vi "imp_test_v7_2encoder.vi"() -> ()   [LabVIEW 2014]
uses:
  <vilib>/LabVIEW Targets/FPGA/cRIO/shared/nicrio_ModuleControls/nicrio_cRIO-9237_DataRatesRing.ctl
  <vilib>/LabVIEW Targets/FPGA/cRIO/shared/nicrio_ModuleControls/nicrio_cRIO-9237_ExcitationVoltageRing.ctl
  <vilib>/rvi/FXPMathLib/FxpSinAndCos/subVIs/nifxpmath_SinAndCos_SimConfig.ctl
  <vilib>/rvi/Emulation/niFpgaGetClockAttributes.vi
  <vilib>/rvi/Emulation/niFpgaSctlEmulationGetInTimedLoop.vi
  <vilib>/rvi/Emulation/niFpgaEmulationReportErrorSimple.vi
  <vilib>/rvi/Emulation/niFpgaProcessEmulError.vi
  <vilib>/rvi/interface/RandomDataEmulation/nirviRandomDataMultiElementFPGAFIFO.vi
  <instcachedir>/0/nirviRandomDataMultiElementFPGAFIFO_AD0CFC12EF974623A9C2E4184BC062B2.lvgen/nirviRandomDataMultiElementFPGAFIFO_AD0CFC12EF974623A9C2E4184BC062B2_023.vi
  <vilib>/rvi/interface/RandomDataEmulation/niFpgaRandomDataHandleErrors.vi
  <vilib>/rvi/Emulation/niFpgaCriticalErrorInLSC.vi
  <vilib>/rvi/eio/common/nirviEmuTemplateMethod_errors.vi
  <vilib>/rvi/FXPMathLib/FxpSinAndCos/simVIs/DllFxpSinAndCosTemp_sub.vi
  <vilib>/rvi/eio/common/nirviEmuTemplatePropertySet_errors.vi
  <vilib>/rvi/DataTransferAndStorage/Container/XNode/niFpgaContainer.xnode
  <vilib>/rvi/interface/RandomDataEmulation/nirviRandomDataFpgaMultiElementTemplate.vi
  <vilib>/eio/EIONode/EIONode.xnode
  <vilib>/rvi/FXPMathLib/FxpMul/XNode/nifxpmath_Multiplier.xnode
  <vilib>/rvi/FXPMathLib/FxpSinAndCos/XNode/nifxpmath_SinAndCos.xnode
  <vilib>/rvi/Analysis/measure/butterworth/XNode/niFpgaButterworthFilter.xnode
  <vilib>/rvi/FXPMathLib/FxpSub/XNode/nifxpmath_Sub.xnode
  <vilib>/rvi/FXPMathLib/FxpAdd/XNode/nifxpmath_Add.xnode
  <vilib>/eio/EIOPropertyNode/EIOPropertyNode.xnode
  <vilib>/rvi/eio/common/nirviEmuTemplatePropertyGet_errors.vi
  <vilib>/rvi/eio/common/nirviEmuTemplatePropertyGet_noerrors.vi
  <vilib>/rvi/eio/common/nirviEmuTemplatePropertySet_noerrors.vi
  <vilib>/rvi/FXPMathLib/sim/FxpSim.dll
panel:
  out "Encoder Position":i32
  out "rad_y (NrTheta)":fxp<+/-,33,20>
  out "D_y (mm)":fxp<+/-,32,7>
  in  "Encoder select":i16(ring) items=["Encoder", "Mag. encoder"]
  in  "Mag encoder coeff.":fxp<+/-,32,14>
  in  "Strain selection_y":i16(ring) items=["Raw", "Avg.8", "Avg.8 w. filter"]
  in  "Belt_oy":fxp<+/-,7,7>
  in  "Belt_my":fxp<+/-,6,6>
  out "Fp_dc":fxp<+/-,32,10>
  out "Fy_dc":fxp<+/-,32,10>
  in  "Zero_y":bool
  in  "Zero_p":bool
  in  "S/F coeff_p":fxp<+/-,25,-10>
  in  "S/F coeff_y":fxp<+/-,25,-10>
  out "Force_p":fxp<+/-,32,10>
  in  "Strain selection_p":i16(ring) items=["Raw", "Avg.8", "Avg.8 w. filter"]
  out "Strain_p (Avg8 w. f)":fxp<+/-,36,8>
  in  "Strain_p Avg.8 coeff.":i32[](array[numeric])=[946630756, 63555534]
  out "Strain_p (Avg8)":fxp<+/-,36,4>
  out "Raw Strain_p":fxp<+/-,36,4>
  out "Mod6/AI3":fxp<+/-,36,4>
  in  "Strain gage reset_p":bool
  out "rad_ym":fxp<+/-,33,20>
  out "D_ym":fxp<+/-,32,7>
  out "encoder position_ym":i32
  in  "Encoder reset_p":bool
  out "Strain_y (Avg8 w. f)":fxp<+/-,36,8>
  in  "Strain_y Avg8 coeff.":i32[](array[numeric])=[-898916953, 1957103773, 3888751]
  out "Dyr_for":fxp<+/-,22,7>
  in  "Command_y":i16(ring) items=["Step", "Sine"]
  out "Strain_y (Avg8)":fxp<+/-,36,4>
  out "vb_y":fxp<+/-,38,8>
  out "va_y":fxp<+/-,38,8>
  out "fyt_d":fxp<+/-,36,18>
  out "Fr_y":fxp<+/-,32,10>
  in  "Bv_y":fxp<+/-,22,8>
  out "Dy_error_dd":fxp<+/-,36,16>
  out "Dy_error_d":fxp<+/-,33,8>
  in  "Kv_y":fxp<+/-,22,8>
  out "Dy_error":fxp<+/-,22,7>
  out "Dyr_sin_dd":fxp<+/-,35,20>
  out "Dyr_sin_d":fxp<+/-,33,15>
  out "Sin omega_y":fxp<+/-,34,9>
  out "Dyr_sin":fxp<+/-,22,7>
  in  "Sin offset_y":fxp<+/-,22,7>
  in  "Sin magnitude_y":fxp<+/-,21,6>
  out "Time now(s)":fxp<+,52,14>
  in  "Sin wave freq._y (Hz)":fxp<+/-,32,6>
  in  "Dyr_step":fxp<+/-,22,7>
  in  "Drive mode":i16(ring) items=["Backward", "Forward"]
  out "Dy_dd":fxp<+/-,36,25>
  in  "Dy_dd coeff.":i32[](array[numeric])=[946630756, 63555534]
  out "dFy_PID":fxp<+/-,36,18>
  in  "dFy_PID coeff.":i32[](array[numeric])=[946630756, 63555534]
  out "fyt_i":fxp<+/-,36,16>
  out "Fy_PID":fxp<+/-,36,16>
  in  "fy_tolorance":fxp<+,22,6>
  in  "Ki_y":fxp<+/-,36,9>
  in  "Kd_y":fxp<+/-,36,9>
  out "fy_tilde":fxp<+/-,32,10>
  in  "Kp_y":fxp<+/-,36,9>
  out "vq_y_F":fxp<+/-,20,5> format="%.57g"
  out "vd_y_F":fxp<+/-,20,5>
  in  "dFy_add":bool
  in  "Stop motor_y":bool
  out "Dy_d (mm/s)":fxp<+/-,36,11>
  out "omega_y (rad/s)":fxp<+/-,20,9>
  in  "mt0_omega_y":u32
  out "mt_omega_y":u32
  out "rad_y":fxp<+/-,33,20>
  out "D_y":fxp<+/-,32,7>
  out "encoder position_y":i32
  in  "Encoder reset_y":bool
  in  "Ini coe.":bool
  out "Loop rate (kHz)":fxp<+/-,36,7>
  out "Force_y":fxp<+/-,32,10>
  out "Raw Strain_y":fxp<+/-,36,4>
  in  "Strain gage reset_y":bool
  in  "Stop (Strain)":bool
  out "Mod6/AI2":fxp<+/-,36,4>
  in  "Excitation Voltage":T1 items=["2.5 Volts", "3.3 Volts", "5.0 Volts", "10.0 Volts", "External Excitation"]
  in  "Data Rate":T2=1 items=["50.000 kS/s (NI 9237)"=1, "25.000 kS/s (NI 9237)"=2, "16.667 kS/s (NI 9237)"=3, "12.500 kS/s (NI 9237)"=4, "10.000 kS/s (NI 9237)"=5, "8.333 kS/s (NI 9237)"=6, "7.143 kS/s (NI 9237)"=7, "6.250 kS/s (NI 9237)"=8, "5.556 kS/s (NI 9237)"=9, "5.000 kS/s (NI 9237)"=10, "4.545 kS/s (NI 9237)"=11, "4.167 kS/s (NI 9237)"=12, "3.846 kS/s (NI 9237)"=13, "3.571 kS/s (NI 9237)"=14, "3.333 kS/s (NI 9237)"=15, "3.125 kS/s (NI 9237)"=16, "2.941 kS/s (NI 9237)"=17, "2.778 kS/s (NI 9237)"=18, "2.632 kS/s (NI 9237)"=19, "2.500 kS/s (NI 9237)"=20, "2.381 kS/s (NI 9237)"=21, "2.273 kS/s (NI 9237)"=22, "2.174 kS/s (NI 9237)"=23, "2.083 kS/s (NI 9237)"=24, "2.000 kS/s (NI 9237)"=25, "1.923 kS/s (NI 9237)"=26, "1.852 kS/s (NI 9237)"=27, "1.786 kS/s (NI 9237)"=28, "1.724 kS/s (NI 9237)"=29, "1.667 kS/s (NI 9237)"=30, "1.613 kS/s (NI 9237)"=31]
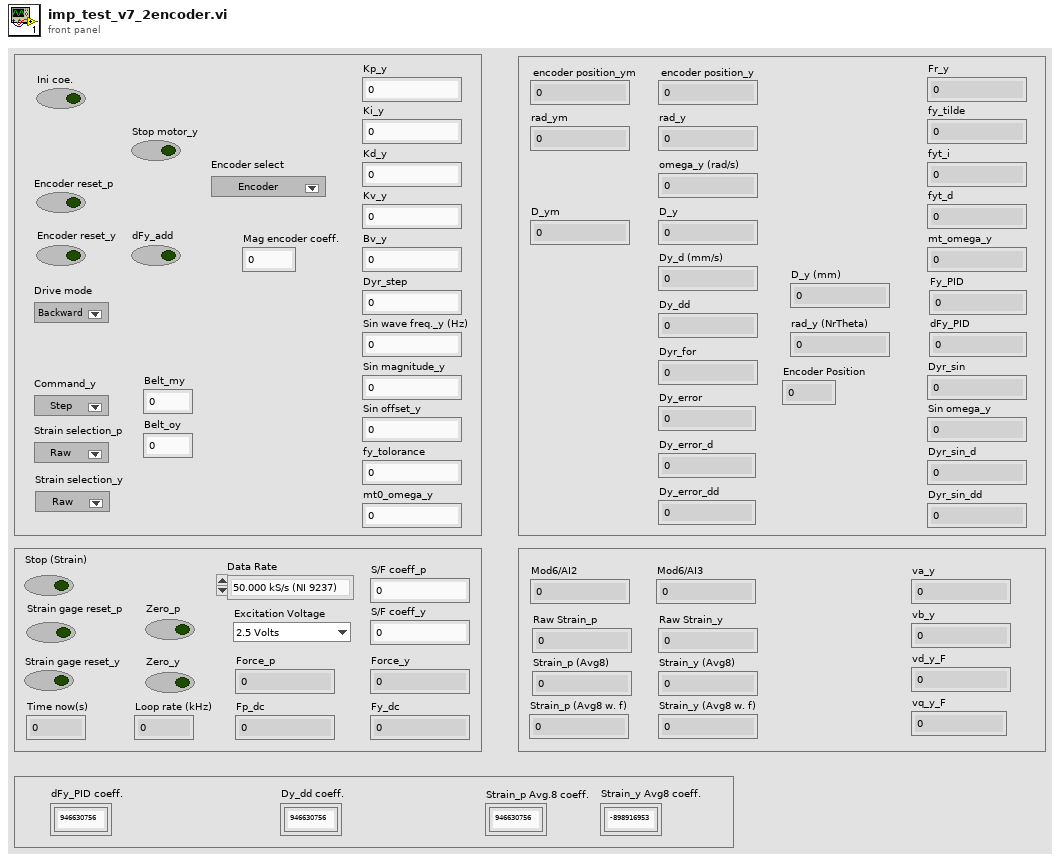
[diagram p1: front panel]
types:
  T1 = typedef "nicrio_cRIO-9237_ExcitationVoltageRing.ctl" = u8
  T2 = typedef "nicrio_cRIO-9237_DataRatesRing.ctl" = u8
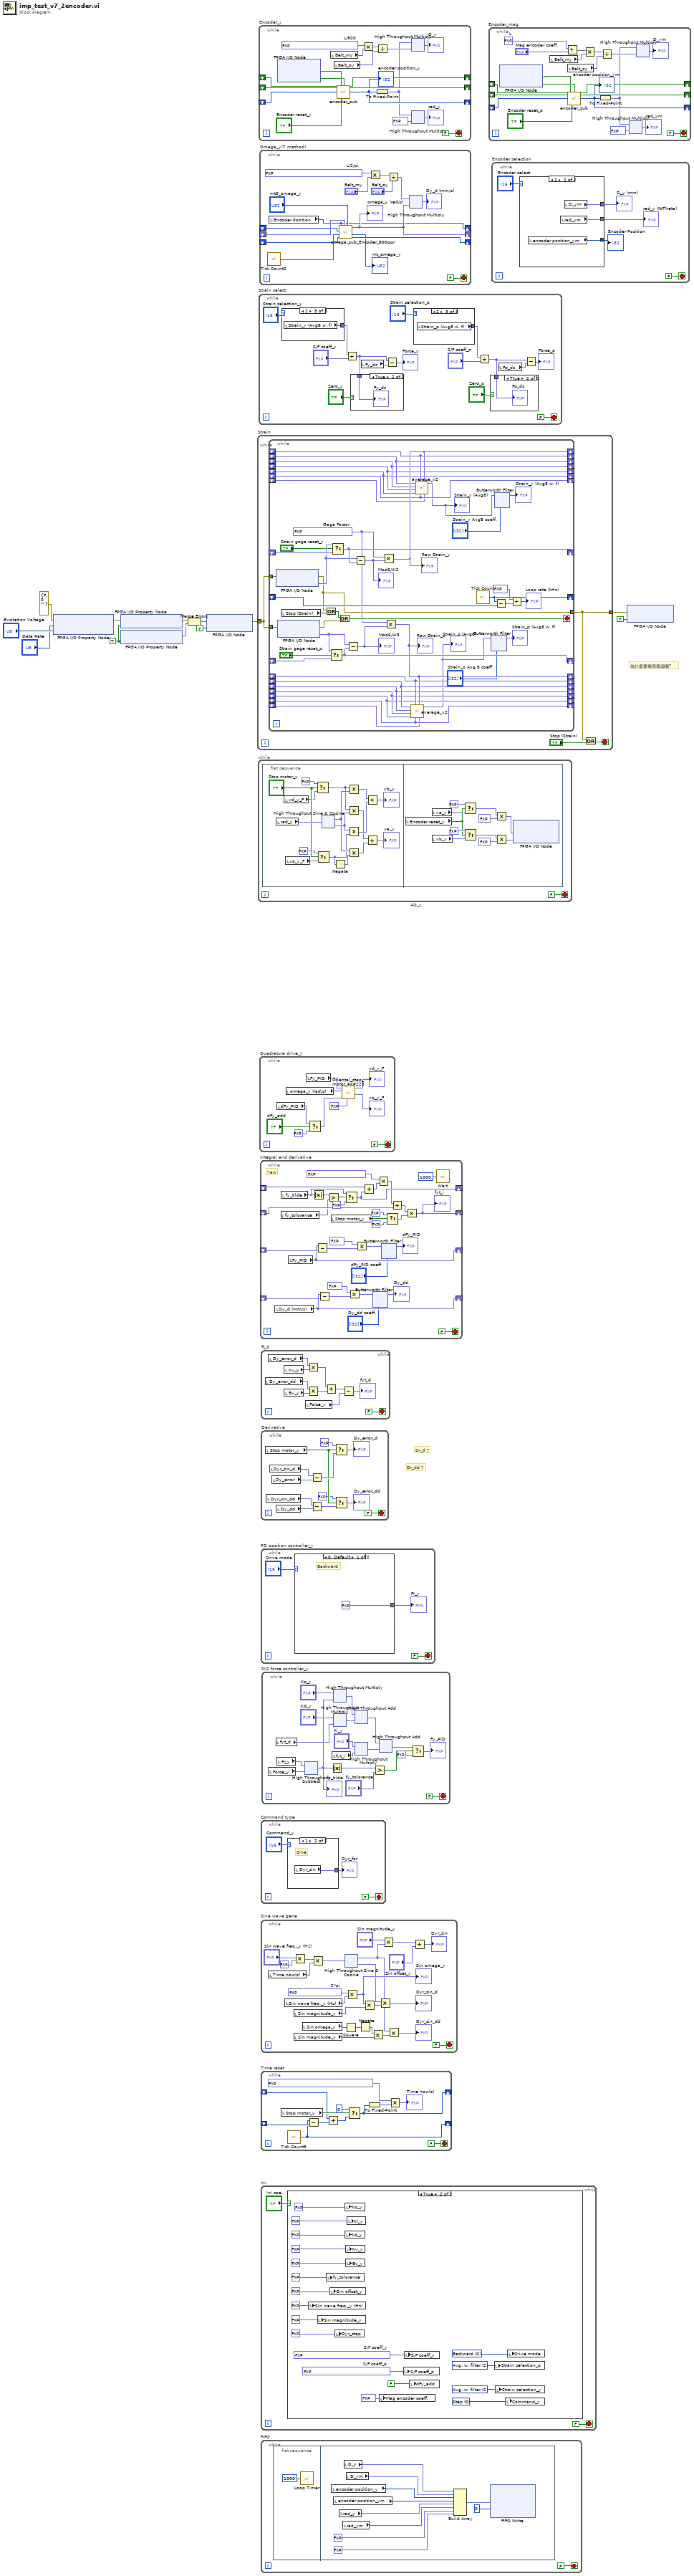
[diagram p0: block diagram]
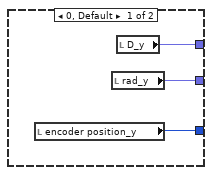
[diagram p2: hidden frame]
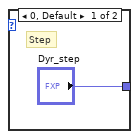
[diagram p3: hidden frame]
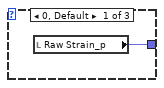
[diagram p6: hidden frame]
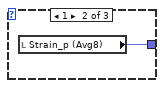
[diagram p7: hidden frame]
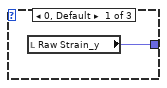
[diagram p8: hidden frame]
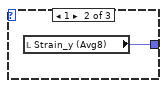
[diagram p9: hidden frame]
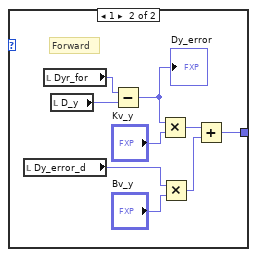
[diagram p10: hidden frame]
diagram:
  w5 = TRUE ("Half-Bridge Enable")
  # "為什麼要寫兩個迴圈?"
  # "Dr_dd ?"
  # "Dr_d ?"
  n1 = xnode "FPGA I/O Property Node"("error in"=errorcluster {"status"=FALSE, "code"=0, "source"=""}, "Data Rate"="Data Rate", "Excitation Voltage"="Excitation Voltage") -> ("error out"=w10:errorcluster)  [unwired: 1 in, 1 out]
  n2 = xnode "FPGA I/O Property Node"("error in"=w10, "Half-Bridge Enable"=w5) -> ("error out"=w3:errorcluster)  [unwired: 1 in, 1 out]
  n3 = xnode "FPGA I/O Property Node"("Half-Bridge Enable"=w5) -> ("error out"=w2:errorcluster)  [unwired: 2 in, 1 out]
  n4 = Merge Errors(w3, w2) -> (w4:errorcluster)
  n5 = xnode "FPGA I/O Node"("error in"=w4, "Mod6/Start"=TRUE) -> ("error out"=w8:errorcluster)  [unwired: 1 in, 1 out]
  n6 = while "Strain" {
    tunnel: w8 -> [w15]
    tunnel: [w13] -> w1
    stop <- w14 stop-if-true
    n7 = while {
      tunnel: w15 -> [w61]
      tunnel: [w34] -> w13
      shift-right: [w58] -> _
      shift-left: _ -> [w59]
      shift-right: [w54] -> _
      shift-left: _ -> [w55]
      shift-right: [w49] -> _
      shift-left: _ -> [w48]
      shift-right: [w48] -> _
      shift-left: _ -> [w47]
      shift-right: [w47] -> _
      shift-left: _ -> [w46]
      shift-right: [w46] -> _
      shift-left: _ -> [w45]
      shift-right: [w45] -> _
      shift-left: _ -> [w44]
      shift-right: [w44] -> _
      shift-left: _ -> [w43]
      shift-right: [w43] -> _
      shift-left: _ -> [w42]
      tunnel: w15 -> [w38]
      shift-right: [w31] -> _
      shift-left: _ -> [w32]
      shift-right: [w27] -> _
      shift-left: _ -> [w26]
      shift-right: [w26] -> _
      shift-left: _ -> [w25]
      shift-right: [w25] -> _
      shift-left: _ -> [w24]
      shift-right: [w24] -> _
      shift-left: _ -> [w23]
      shift-right: [w23] -> _
      shift-left: _ -> [w22]
      shift-right: [w22] -> _
      shift-left: _ -> [w21]
      shift-right: [w21] -> _
      shift-left: _ -> [w20]
      stop <- w35 stop-if-true
      w29 = fxp<+,20,2> 2.115001678466797  # Gage Factor
      n8 = xnode "FPGA I/O Node"("error in"=w61) -> ("error out"=w34:errorcluster, "Mod6/AI2"=w56:fxp<+/-,24,-4>)  [unwired: 1 in, 1 out]
      n9 = xnode "FPGA I/O Node"("error in"=w38) -> ("error out"=w36:errorcluster, "Mod6/AI3"=w30:fxp<+/-,24,-4>)  [unwired: 1 in, 1 out]
      n10 = local read "Stop (Strain)"() -> (w60:bool)
      n11 = Or(x=w34, y=w60) -> (x .or. y?=w37:bool)
      n12 = Select(t=w30, s="Strain gage reset_p", f=w32) -> (s? t:f=w31:fxp<+/-,24,-4>)
      n13 = Select(t=w56, s="Strain gage reset_y", f=w59) -> (s? t:f=w58:fxp<+/-,24,-4>)
      n14 = Or(x=w37, y=w36) -> (x .or. y?=w35:bool)
      n15 = Subtract(x=w30, y=w31) -> (x-y=w28:fxp<+/-,30,-3>)
      "Mod6/AI3" <- w28
      n16 = Subtract(x=w56, y=w58) -> (x-y=w57:fxp<+/-,30,-3>)
      "Mod6/AI2" <- w57
      n17 = Multiply(x=w29, y=w57) -> (x*y=w49:fxp<+/-,41,6>)
      "Raw Strain_y" <- w49
      n18 = Multiply(x=w29, y=w28) -> (x*y=w27:fxp<+/-,50,-1>)
      "Raw Strain_p" <- w27
      n19 = call "average_v2.vi"("Numeric 8"=w20, "Numeric"=w27, "Numeric 7"=w21, "Numeric 2"=w26, "Numeric 6"=w22, "Numeric 5"=w23, "Numeric 4"=w24, "Numeric 3"=w25) -> ("Mean (8pt)"=w19:fxp<+/-,32,4>)  [unwired: 1 in, 2 out]
      "Strain_p (Avg8)" <- w19
      n20 = call "average_v2.vi"("Numeric 8"=w42, "Numeric"=w49, "Numeric 7"=w43, "Numeric 2"=w48, "Numeric 6"=w44, "Numeric 5"=w45, "Numeric 4"=w46, "Numeric 3"=w47) -> ("Mean (8pt)"=w41:fxp<+/-,32,4>)  [unwired: 1 in, 2 out]
      "Strain_y (Avg8)" <- w41
      n21 = call "Tick Count"() -> ("Tick Count(uSec)"=w54:u32)
      n22 = xnode "Butterworth Filter"("input data"=w19, "scaled coefficients"="Strain_p Avg.8 coeff.") -> ("output data"=→"Strain_p (Avg8 w. f)":fxp<+/-,36,8>)  [unwired: 1 in]
      n23 = xnode "Butterworth Filter"("input data"=w41, "scaled coefficients"="Strain_y Avg8 coeff.") -> ("output data"=→"Strain_y (Avg8 w. f)":fxp<+/-,32,4>)  [unwired: 1 in]
      n24 = Subtract(x=w54, y=w55) -> (x-y=w52:fxp<+/-,32,16>)
      n25 = Divide(x=fxp<+,7,10> 1000.0, y=w52) -> (x/y=→"Loop rate (kHz)":fxp<+/-,40,27>)
    }
    n26 = Or(x=w13, y="Stop (Strain)") -> (x .or. y?=w14:bool)
  }
  n27 = while "AO_y" {
    stop <- FALSE stop-if-true
    n28 = flat-sequence {
      frame #0 {
        n29 = local read "rad_y"() -> (w95:fxp<+/-,33,20>)
        n30 = local read "vd_y_F"() -> (w93:fxp<+/-,20,5>)
        n31 = local read "vq_y_F"() -> (w92:fxp<+/-,20,5>)
        n32 = Select(t=fxp<+/-,20,5> 0.0, s="Stop motor_y", f=w93) -> (s? t:f=w87:fxp<+/-,20,5>)
        n33 = Select(t=fxp<+/-,20,5> 0.0, s="Stop motor_y", f=w92) -> (s? t:f=w86:fxp<+/-,20,5>)
        n34 = xnode "High Throughput Sine & Cosine"("x (pi)"=w95) -> ("sin(x)"=w89:fxp<+/-,17,2>, "cos(x)"=w88:fxp<+/-,17,2>)
        n35 = Negate(x=w86) -> (-x=w85:fxp<+/-,21,6>)
        n36 = Multiply(x=w87, y=w89) -> (x*y=w84:fxp<+/-,37,7>)
        n37 = Multiply(x=w87, y=w88) -> (x*y=w82:fxp<+/-,37,7>)
        n38 = Multiply(x=w88, y=w86) -> (x*y=w83:fxp<+/-,37,7>)
        n39 = Multiply(x=w89, y=w85) -> (x*y=w81:fxp<+/-,36,6>)
        n40 = Add(x=w84, y=w83) -> (x+y=→"vb_y":fxp<+/-,38,8>)
        n41 = Add(x=w82, y=w81) -> (x+y=→"va_y":fxp<+/-,37,7>)
      }
      frame #1 {
        n42 = local read "Encoder reset_y"() -> (w128:bool)
        n43 = local read "va_y"() -> (w127:fxp<+/-,38,8>)
        n44 = local read "vb_y"() -> (w126:fxp<+/-,38,8>)
        n45 = Select(t=fxp<+,2,2> 3.0, s=w128, f=w127) -> (s? t:f=w132:fxp<+/-,38,8>)
        n46 = Select(t=fxp<+,1,1> 0.0, s=w128, f=w126) -> (s? t:f=w131:fxp<+/-,38,8>)
        n47 = Multiply(x=w132, y=fxp<+/-,1,0> -0.5) -> (x*y=w135:fxp<+/-,39,8>)
        n48 = Multiply(x=w131, y=fxp<+/-,1,0> -0.5) -> (x*y=w136:fxp<+/-,37,6>)
        n49 = xnode "FPGA I/O Node"("Mod8/AO2"=w135, "Mod8/AO3"=w136) -> ()  [unwired: 2 in, 2 out]
      }
    }
  }
  n50 = while "Strain select." {
    stop <- FALSE stop-if-true
    n51 = case shown="2" "Strain selection_y" {
      tunnel: [w157 w158 w159] -> w151
      frame 0, Default {
        n52 = local read "Raw Strain_y"() -> (w157:fxp<+/-,36,4>)
      }
      frame 1 {
        n53 = local read "Strain_y (Avg8)"() -> (w158:fxp<+/-,36,4>)
      }
      frame 2 {
        n54 = local read "Strain_y (Avg8 w. f)"() -> (w159:fxp<+/-,36,8>)
      }
    }
    n55 = Divide(x=w151, y="S/F coeff_y") -> (x/y=w144:fxp<+/-,32,10>)
    n56 = case shown="True" "Zero_y" {
      tunnel: w144 -> [_ w153]
      frame False {
      }
      frame True {
        "Fy_dc" <- w153
      }
    }
    n57 = local read "Fy_dc"() -> (w145:fxp<+/-,32,10>)
    n58 = Subtract(x=w144, y=w145) -> (x-y=→"Force_y":fxp<+/-,33,11>)
    n59 = case shown="2" "Strain selection_p" {
      tunnel: [w154 w155 w156] -> w149
      frame 0, Default {
        n60 = local read "Raw Strain_p"() -> (w154:fxp<+/-,36,4>)
      }
      frame 1 {
        n61 = local read "Strain_p (Avg8)"() -> (w155:fxp<+/-,36,4>)
      }
      frame 2 {
        n62 = local read "Strain_p (Avg8 w. f)"() -> (w156:fxp<+/-,36,8>)
      }
    }
    n63 = Divide(x=w149, y="S/F coeff_p") -> (x/y=w141:fxp<+/-,32,10>)
    n64 = case shown="True" "Zero_p" {
      tunnel: w141 -> [_ w152]
      frame False {
      }
      frame True {
        "Fp_dc" <- w152
      }
    }
    n65 = local read "Fp_dc"() -> (w139:fxp<+/-,32,10>)
    n66 = Subtract(x=w141, y=w139) -> (x-y=→"Force_p":fxp<+/-,33,11>)
  }
  n67 = while "Encoder_y" {
    shift-right: [w175] -> _
    shift-left: _ -> [w176]
    shift-right: [w177] -> _
    shift-left: _ -> [w178]
    shift-right: [w170] -> _
    shift-left: _ -> [w174]
    stop <- FALSE stop-if-true
    w164 = fxp<+/-,20,-5> 0.002499997615814209  # L/800
    n68 = xnode "FPGA I/O Node"() -> ("Mod4/DI3"=w173:bool, "Mod4/DI4"=w172:bool)  [unwired: 2 in, 2 out]
    n69 = local read "Belt_my"() -> (w163:fxp<+/-,6,6>)
    n70 = local read "Belt_oy"() -> (w161:fxp<+/-,7,7>)
    n71 = call "encoder_sub.vi"("A_pre"=w176, "B_pre"=w178, "Encoder Position_pre"=w174, "A input"=w173, "Encoder Position Reset"="Encoder reset_y", "B input"=w172) -> ("A"=w175:bool, "B"=w177:bool, "Encoder Position (Counts)"=w170:i32)  [unwired: 19 in]
    "encoder position_y" <- w170
    n72 = Multiply(x=w164, y=w163) -> (x*y=w162:fxp<+/-,26,1>)
    n73 = To Fixed-Point(number=w170) -> (fixed-point=w169:fxp<+/-,32,32>)  [unwired: 1 in]
    n74 = Divide(x=w162, y=w161) -> (x/y=w160:fxp<+/-,33,1>)
    n75 = xnode ("High Throughput Multiply")("x"=w169, "y"=w160) -> ("x*y"=→"D_y":fxp<+/-,64,33>)
    n76 = xnode ("High Throughput Multiply")("x"=w169, "y"=fxp<+/-,16,1> 0.125) -> ("x*y"=→"rad_y":fxp<+/-,48,33>)
  }
  n77 = while "Omega_y(T method)" {
    shift-right: [w185] -> _
    shift-left: _ -> [w186]
    shift-right: [w188] -> _
    shift-left: _ -> [w190]
    shift-right: [w192] -> _
    shift-left: _ -> [w193]
    stop <- FALSE stop-if-true
    w183 = fxp<+/-,32,0> 0.3183098859153688  # L/2/pi
    n78 = call "Tick Count2"() -> ("Tick Count(Ticks)"=w194:u32)
    n79 = local read "Encoder Position"() -> (w185:i32)
    n80 = call "omega_sub_Encoder_800ppr.vi"("mt0"="mt0_omega_y", "omega_pre"=w190, "ticks_m_pre"=w193, "ticks"=w194, "count_pre"=w186, "count"=w185) -> ("ticks_m"=w192:u32, "mt"=→"mt_omega_y":u32, "omega"=w188:fxp<+/-,20,9>)  [unwired: 3 in]
    "omega_y (rad/s)" <- w188
    n81 = Multiply(x=w183, y="Belt_my") -> (x*y=w181:fxp<+/-,38,6>)
    n82 = Divide(x=w181, y="Belt_oy") -> (x/y=w179:fxp<+/-,20,1>)
    n83 = xnode ("High Throughput Multiply")("x"=w179, "y"=w188) -> ("x*y"=→"Dy_d (mm/s)":fxp<+/-,40,10>)
  }
  n84 = while "Quadrature drive_y" {
    stop <- FALSE stop-if-true
    n85 = local read "dFy_PID"() -> (w196:fxp<+/-,36,18>)
    n86 = local read "omega_y (rad/s)"() -> (w204:fxp<+/-,20,9>)
    n87 = local read "Fy_PID"() -> (w197:fxp<+/-,36,16>)
    n88 = Select(t=w196, s="dFy_add", f=fxp<+,1,1> 0.0) -> (s? t:f=w200:fxp<+/-,36,18>)
    n89 = call "Oriental_step_motor_PKP225.vi"("F_Threshold"=fxp<+,12,12> 10.0, "dFmr"=w200, "omega"=w204, "Fmr"=w197) -> ("vq_F"=→"vq_y_F":fxp<+/-,20,5>, "vd_F"=→"vd_y_F":fxp<+/-,20,5>)  [unwired: 6 in]
  }
  n90 = while "Integral and derivative" {
    shift-right: [w229] -> _
    shift-left: _ -> [w228]
    shift-right: [w221] -> _
    shift-left: _ -> [w220]
    shift-right: [w231] -> _
    shift-left: _ -> [w232]
    shift-right: [w211] -> _
    shift-left: _ -> [w210]
    stop <- FALSE stop-if-true
    # "Yaw"
    n91 = local read "Dy_d (mm/s)"() -> (w211:fxp<+/-,36,11>)
    n92 = local read "fy_tolorance"() -> (w207:fxp<+,22,6>)
    n93 = local read "fy_tilde"() -> (w233:fxp<+/-,32,10>)
    n94 = local read "Fy_PID"() -> (w231:fxp<+/-,36,16>)
    n95 = Absolute Value(x=w233) -> (abs(x)=w235:fxp<+,32,10>)
    n96 = Subtract(x=w231, y=w232) -> (x-y=w219:fxp<+/-,37,17>)
    n97 = Subtract(x=w211, y=w210) -> (x-y=w213:fxp<+/-,36,11>)
    n98 = Greater?(x=w235, y=w207) -> (0:w236:bool)
    n99 = local read "Stop motor_y"() -> (w222:bool)
    n100 = Select(t=w233, s=w236, f=fxp<+/-,33,11> 0.0) -> (s? t:f=w229:fxp<+/-,33,11>)
    n101 = Multiply(x=fxp<+,7,10> 1000.0, y=w213) -> (x*y=w212:fxp<+/-,36,21>)
    n102 = Multiply(x=fxp<+,7,10> 1000.0, y=w219) -> (x*y=w216:fxp<+/-,32,18>)
    n103 = Add(x=w228, y=w229) -> (x+y=w234:fxp<+/-,34,12>)
    n104 = xnode "Butterworth Filter"("input data"=w212, "scaled coefficients"="Dy_dd coeff.") -> ("output data"=→"Dy_dd":fxp<+/-,36,25>)  [unwired: 1 in]
    n105 = Multiply(x=fxp<+/-,30,12> 0.000499725341796875, y=w234) -> (x*y=w227:fxp<+/-,34,10>)
    n106 = xnode "Butterworth Filter"("input data"=w216, "scaled coefficients"="dFy_PID coeff.") -> ("output data"=→"dFy_PID":fxp<+/-,36,22>)  [unwired: 1 in]
    n107 = Select(t=fxp<+,1,1> 0.0, s=w222, f=fxp<+,1,1> 1.0) -> (s? t:f=w225:fxp<+,1,1>)
    n108 = Add(x=w227, y=w220) -> (x+y=w226:fxp<+/-,36,16>)
    n109 = Multiply(x=w226, y=w225) -> (x*y=w221:fxp<+/-,34,18>)
    "fyt_i" <- w221
    n110 = call "Wait"("Count(uSec)"=u32 1000) -> ()  [unwired: 1 out]
  }
  n111 = while "PD position controller_y" {
    stop <- FALSE stop-if-true
    n112 = case shown="0, Default" "Drive mode" {
      tunnel: [fxp<+/-,62,19> 0.0 w259] -> w255
      frame 0, Default {
        # "Backward"
      }
      frame 1 {
        # "Forward"
        n113 = local read "Dy_error_d"() -> (w261:fxp<+/-,33,8>)
        n114 = local read "Dyr_for"() -> (w258:fxp<+/-,22,7>)
        n115 = local read "D_y"() -> (w266:fxp<+/-,32,7>)
        n116 = Subtract(x=w258, y=w266) -> (x-y=w265:fxp<+/-,33,8>)
        "Dy_error" <- w265
        n117 = Multiply(x=w265, y="Kv_y") -> (x*y=w263:fxp<+/-,54,15>)
        n118 = Multiply(x=w261, y="Bv_y") -> (x*y=w260:fxp<+/-,55,16>)
        n119 = Add(x=w263, y=w260) -> (x+y=w259:fxp<+/-,55,16>)
      }
    }
    "Fr_y" <- w255
  }
  n120 = while "Command type" {
    stop <- FALSE stop-if-true
    n121 = case shown="1" "Command_y" {
      tunnel: ["Dyr_step" w271] -> w268
      frame 0, Default {
        # "Step"
      }
      frame 1 {
        # "Sine"
        n122 = local read "Dyr_sin"() -> (w271:fxp<+/-,22,7>)
      }
    }
    "Dyr_for" <- w268
  }
  n123 = while "Sine wave gene" {
    stop <- FALSE stop-if-true
    w286 = fxp<+,20,3> 6.2831878662109375  # 2*pi
    n124 = local read "Time now(s)"() -> (w292:fxp<+,52,14>)
    n125 = local read "Sin wave freq._y (Hz)"() -> (w285:fxp<+/-,32,6>)
    n126 = Multiply(x="Sin wave freq._y (Hz)", y=fxp<+/-,10,3> 2.0) -> (x*y=w293:fxp<+/-,41,9>)
    n127 = local read "Sin magnitude_y"() -> (w283:fxp<+/-,21,6>)
    n128 = local read "Sin magnitude_y"() -> (w276:fxp<+/-,21,6>)
    n129 = local read "Sin omega_y"() -> (w279:fxp<+/-,34,9>)
    n130 = Multiply(x=w293, y=w292) -> (x*y=w291:fxp<+/-,41,19>)
    n131 = Square(x=w279) -> (x^2=w278:fxp<+,34,18>)
    n132 = xnode "High Throughput Sine & Cosine"("x (pi)"=w291) -> ("sin(x)"=w273:fxp<+/-,16,2>, "cos(x)"=w281:fxp<+/-,16,2>)
    n133 = Multiply(x=w286, y=w285) -> (x*y=w284:fxp<+/-,34,9>)
    "Sin omega_y" <- w284
    n134 = Negate(x=w278) -> (-x=w277:fxp<+/-,35,19>)
    n135 = Multiply(x=w284, y=w283) -> (x*y=w282:fxp<+/-,33,15>)
    n136 = Multiply(x=w277, y=w276) -> (x*y=w275:fxp<+/-,34,20>)
    n137 = Multiply(x=w281, y=w282) -> (x*y=→"Dyr_sin_d":fxp<+/-,33,15>)
    n138 = Multiply(x="Sin magnitude_y", y=w273) -> (x*y=w289:fxp<+/-,37,8>)
    n139 = Multiply(x=w273, y=w275) -> (x*y=→"Dyr_sin_dd":fxp<+/-,35,20>)
    n140 = Add(x=w289, y="Sin offset_y") -> (x+y=→"Dyr_sin":fxp<+/-,37,8>)
  }
  n141 = while "Time reset" {
    shift-right: [w335] -> _
    shift-left: _ -> [w336]
    shift-right: [w330] -> _
    shift-left: _ -> [w331]
    stop <- FALSE stop-if-true
    n142 = local read "Stop motor_y"() -> (w337:bool)
    n143 = call "Tick Count3"() -> ("Tick Count(uSec)"=w335:u32)
    n144 = Subtract(x=w335, y=w336) -> (x-y=w334:u32)
    n145 = Add(x=w331, y=w334) -> (x+y=w333:u32)
    n146 = Select(t=u32 0, s=w337, f=w333) -> (s? t:f=w330:u32)
    n147 = To Fixed-Point(number=w330) -> (fixed-point=w329:fxp<+,32,32>)  [unwired: 1 in]
    n148 = Multiply(x=fxp<+,20,-18> 1.0000003385357559e-06, y=w329) -> (x*y=→"Time now(s)":fxp<+,52,14>)
  }
  n149 = while "Ini" {
    stop <- FALSE stop-if-true
    n150 = case shown="True" "Ini coe." {
      frame False {
      }
      frame True {
        w341 = i16 2 items=["Raw", "Avg.", "Avg. w. filter"] ("Strain selection_p")
        w342 = i16 0 items=["Step", "Sine"] ("Command_y")
        w343 = i16 2 items=["Raw", "Avg.", "Avg. w. filter"] ("Strain selection_y")
        w345 = fxp<+/-,25,-10> 5.851034075021744e-07  # S/F coeff_p
        w344 = fxp<+/-,25,-10> 1.0477961041033268e-06  # S/F coeff_y
        w351 = i16 0 items=["Backward", "Forward"] ("Drive mode")
        n151 = local write "Sin wave freq._y (Hz)"(fxp<+/-,32,6> 1.0 ("Sin wave freq. (Hz)")) -> ()
        n152 = local write "Sin magnitude_y"(fxp<+/-,22,7> 5.0 ("Sin magnitude")) -> ()
        n153 = local write "fy_tolorance"(fxp<+,22,6> 5.0 ("f_tolorance")) -> ()
        n154 = local write "Sin offset_y"(fxp<+/-,38,9> 0.0 ("Sin offset")) -> ()
        n155 = local write "Dyr_step"(fxp<+/-,22,7> 0.0 ("Dr")) -> ()
        n156 = local write "Kp_y"(fxp<+/-,36,9> 30.0 ("Kp")) -> ()
        n157 = local write "Kd_y"(fxp<+/-,36,9> 0.0 ("Kd")) -> ()
        n158 = local write "Kv_y"(fxp<+/-,22,8> 0.0 ("Kv")) -> ()
        n159 = local write "Bv_y"(fxp<+/-,22,8> 0.0 ("Bv")) -> ()
        n160 = local write "Ki_y"(fxp<+/-,36,9> 0.0 ("Ki")) -> ()
        n161 = local write "Mag encoder coeff."(fxp<+/-,32,14> 4096.0 ("Mag encoder coeff.")) -> ()
        n162 = local write "S/F coeff_p"(w345) -> ()
        n163 = local write "S/F coeff_y"(w344) -> ()
        n164 = local write "dFy_add"(FALSE ("dF_add")) -> ()
        n165 = local write "Strain selection_p"(w341) -> ()
        n166 = local write "Strain selection_y"(w343) -> ()
        n167 = local write "Command_y"(w342) -> ()
        n168 = local write "Drive mode"(w351) -> ()
      }
    }
  }
  n169 = while "FIFO" {
    stop <- FALSE stop-if-true
    n170 = flat-sequence {
      frame #0 {
        n171 = call "Loop Timer"("Count(uSec)"=u32 1000) -> ()  [unwired: 1 out]
      }
      frame #1 {
        n172 = local read "encoder position_y"() -> (w367:i32)
        n173 = local read "encoder position_ym"() -> (w366:i32)
        n174 = local read "rad_y"() -> (w363:fxp<+/-,33,20>)
        n175 = local read "rad_ym"() -> (w364:fxp<+/-,33,20>)
        n176 = local read "D_y"() -> (w369:fxp<+/-,32,7>)
        n177 = local read "D_ym"() -> (w368:fxp<+/-,32,7>)
        n178 = Build Array(w369, w368, w367, w366, w363, w364, fxp<+/-,43,11> 0.0 ("element"), fxp<+/-,43,11> 0.0 ("element")) -> (w362:fxp<+/-,64,32>[])
        n179 = xnode ("FIFO Write")("Element"=w362, "Timeout"=0) -> ()  [unwired: 1 in, 2 out]
      }
    }
  }
  n180 = while "ft_d" {
    stop <- FALSE stop-if-true
    n181 = local read "Dy_error_dd"() -> (w376:fxp<+/-,36,16>)
    n182 = local read "Dy_error_d"() -> (w378:fxp<+/-,33,8>)
    n183 = local read "Kv_y"() -> (w379:fxp<+/-,22,8>)
    n184 = local read "Bv_y"() -> (w377:fxp<+/-,22,8>)
    n185 = local read "Force_y"() -> (w372:fxp<+/-,32,10>)
    n186 = Multiply(x=w378, y=w379) -> (x*y=w374:fxp<+/-,55,16>)
    n187 = Multiply(x=w376, y=w377) -> (x*y=w375:fxp<+/-,58,24>)
    n188 = Add(x=w374, y=w375) -> (x+y=w373:fxp<+/-,63,24>)
    n189 = Subtract(x=w373, y=w372) -> (x-y=→"fyt_d":fxp<+/-,63,24>)
  }
  n190 = while "Derivative" {
    stop <- FALSE stop-if-true
    n191 = local read "Stop motor_y"() -> (w383:bool)
    n192 = local read "Dyr_sin_dd"() -> (w385:fxp<+/-,35,20>)
    n193 = local read "Dyr_sin_d"() -> (w388:fxp<+/-,33,15>)
    n194 = local read "Dy_error"() -> (w389:fxp<+/-,22,7>)
    n195 = local read "Dy_dd"() -> (w386:fxp<+/-,36,25>)
    n196 = Subtract(x=w388, y=w389) -> (x-y=w387:fxp<+/-,34,16>)
    n197 = Subtract(x=w385, y=w386) -> (x-y=w384:fxp<+/-,41,26>)
    n198 = Select(t=fxp<+,1,1> 0.0, s=w383, f=w387) -> (s? t:f=→"Dy_error_d":fxp<+/-,34,16>)
    n199 = Select(t=fxp<+/-,64,49> 0.0, s=w383, f=w384) -> (s? t:f=→"Dy_error_dd":fxp<+/-,64,49>)
  }
  n200 = while "PID force controller_y" {
    stop <- FALSE stop-if-true
    n201 = local read "Force_y"() -> (w409:fxp<+/-,32,10>)
    n202 = local read "fyt_d"() -> (w393:fxp<+/-,36,18>)
    n203 = local read "Fr_y"() -> (w395:fxp<+/-,32,10>)
    n204 = xnode "High Throughput Subtract"("x"=w395, "y"=w409) -> ("x-y"=w408:fxp<+/-,33,11>)
    "fy_tilde" <- w408
    n205 = Absolute Value(x=w408) -> (abs(x)=w399:fxp<+,33,11>)
    n206 = local read "fyt_i"() -> (w394:fxp<+/-,36,16>)
    n207 = xnode ("High Throughput Multiply")("x"="Kp_y", "y"=w408) -> ("x*y"=w406:fxp<+/-,64,20>)
    n208 = xnode ("High Throughput Multiply")("x"="Kd_y", "y"=w393) -> ("x*y"=w405:fxp<+/-,64,27>)
    n209 = xnode ("High Throughput Add")("x"=w406, "y"=w405) -> ("x+y"=w402:fxp<+/-,64,28>)
    n210 = xnode ("High Throughput Multiply")("x"="Ki_y", "y"=w394) -> ("x*y"=w403:fxp<+/-,64,25>)
    n211 = Greater?(x=w399, y="fy_tolorance") -> (0:w397:bool)
    n212 = xnode ("High Throughput Add")("x"=w402, "y"=w403) -> ("x+y"=w401:fxp<+/-,64,29>)
    n213 = Select(t=w401, s=w397, f=fxp<+/-,51,14> 0.0) -> (s? t:f=→"Fy_PID":fxp<+/-,64,29>)
  }
  n214 = while "Encoder_mag" {
    shift-right: [w427] -> _
    shift-left: _ -> [w428]
    shift-right: [w429] -> _
    shift-left: _ -> [w430]
    shift-right: [w423] -> _
    shift-left: _ -> [w431]
    stop <- FALSE stop-if-true
    w411 = fxp<+/-,20,3> 2.0  # L
    n215 = xnode "FPGA I/O Node"() -> ("Mod4/DI0"=w425:bool, "Mod4/DI1"=w426:bool)  [unwired: 2 in, 2 out]
    n216 = local read "Belt_my"() -> (w417:fxp<+/-,6,6>)
    n217 = Divide(x=w411, y="Mag encoder coeff.") -> (x/y=w412:fxp<+/-,32,3>)
    n218 = local read "Belt_oy"() -> (w415:fxp<+/-,7,7>)
    n219 = call "encoder_sub.vi"("A_pre"=w428, "B_pre"=w430, "Encoder Position_pre"=w431, "A input"=w425, "Encoder Position Reset"="Encoder reset_p", "B input"=w426) -> ("A"=w427:bool, "B"=w429:bool, "Encoder Position (Counts)"=w423:i32)  [unwired: 19 in]
    "encoder position_ym" <- w423
    n220 = Multiply(x=w412, y=w417) -> (x*y=w416:fxp<+/-,38,9>)
    n221 = To Fixed-Point(number=w423) -> (fixed-point=w422:fxp<+/-,32,32>)  [unwired: 1 in]
    n222 = Divide(x=w416, y=w415) -> (x/y=w414:fxp<+/-,45,9>)
    n223 = xnode ("High Throughput Multiply")("x"=w422, "y"=fxp<+/-,16,1> 0.125) -> ("x*y"=→"rad_ym":fxp<+/-,48,33>)
    n224 = xnode ("High Throughput Multiply")("x"=w422, "y"=w414) -> ("x*y"=→"D_ym":fxp<+/-,64,41>)
  }
  n225 = while "Encoder selection" {
    stop <- FALSE stop-if-true
    n226 = case shown="1" "Encoder select" {
      tunnel: [w439 w441] -> w434
      tunnel: [w438 w440] -> w433
      tunnel: [w437 w442] -> w435
      frame 0, Default {
        n227 = local read "encoder position_y"() -> (w437:i32)
        n228 = local read "rad_y"() -> (w439:fxp<+/-,33,20>)
        n229 = local read "D_y"() -> (w438:fxp<+/-,32,7>)
      }
      frame 1 {
        n230 = local read "encoder position_ym"() -> (w442:i32)
        n231 = local read "rad_ym"() -> (w441:fxp<+/-,33,20>)
        n232 = local read "D_ym"() -> (w440:fxp<+/-,32,7>)
      }
    }
    "D_y (mm)" <- w433
    "rad_y (NrTheta)" <- w434
    "Encoder Position" <- w435
  }
  n233 = xnode "FPGA I/O Node"("error in"=w1, "Mod6/Stop"=TRUE) -> ()  [unwired: 1 in, 2 out]
